vi "Save Settings to XML.vi"(8 "error in (no error)":errorcluster, 11 "Settings":T1) -> (0 "error out":errorcluster)   [LabVIEW 2019, in "Settings.lvlib"]
doc: "Saves the \"User Specified\" configuration data to an XML file. This is used to remember the users settings between executions."
uses:
  Settings.lvlib
  Cluster - Settings.ctl
  MainController/Cluster - HardwareConfiguration.ctl
  MainController/Cluster - LoggingConfiguration.ctl
  AutoMode/Cluster - AutoModeSettings.ctl
  <vilib>/Utility/xml.llb/Write to XML File(string).vi
  MainController/MainController.lvlib
  AutoMode/AutoMode.lvlib
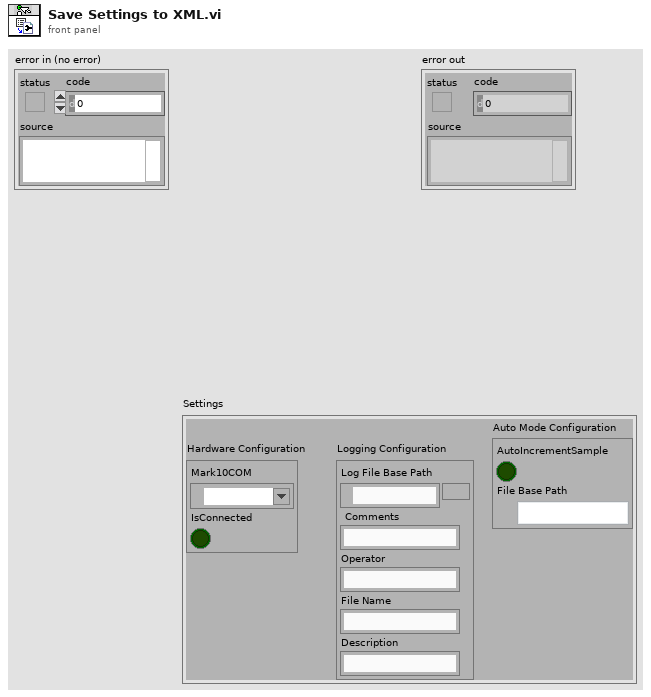
[diagram p1: front panel]
types:
  T1 = typedef "Settings.lvlib/Cluster - Settings.ctl" = cluster{"Hardware Configuration":T2, "Logging Configuration":T3, "Auto Mode Configuration":T4}
  T2 = typedef "MainController.lvlib/Cluster - HardwareConfiguration.ctl" = cluster{"Mark10COM":refnum<visa-resource-name>, "IsConnected":bool}
  T3 = typedef "MainController.lvlib/Cluster - LoggingConfiguration.ctl" = cluster{"Log File Base Path":path, "Comments ":string, "Operator":string, "File Name":string, "Description":string}
  T4 = typedef "AutoMode.lvlib/Cluster - AutoModeSettings.ctl" = cluster{"AutoIncrementSample":bool, "File Base Path":path}
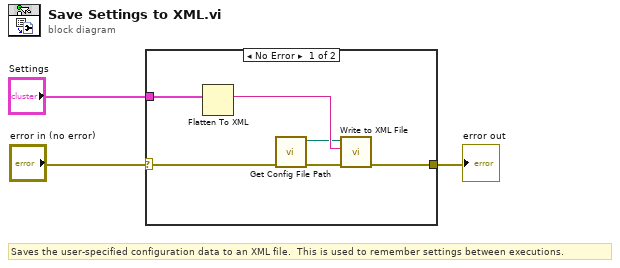
[diagram p0: block diagram]
diagram:
  # "Saves the user-specified configuration data to an XML file.  This is used to remember settings between executions."
  n1 = case shown="No Error" "error in (no error)" {
    selector: "error in (no error)" -> [w5 w10]
    tunnel: [w7 w10] -> w2
    tunnel: "Settings" -> [w9 _]
    frame No Error {
      n2 = Flatten To XML(anything=w9) -> (xml string=w8:string)
      n3 = call "Get Config File Path.vi"("error in (no error)"=w5) -> ("error out"=w4:errorcluster, "XML File Path"=w6:path)  [unwired: 9 in]
      n4 = call-poly <vilib>:"Write to XML File.vi"("error in (no error)"=w4, "XML Input"=w8, "XML File Path"=w6) -> ("error out"=w7:errorcluster)  [unwired: 6 in, 2 out]
    }
    frame Error {
    }
  }
  "error out" <- w2
